vi "Read Comments.vi"(8 "error in (no error)":errorcluster, 11 "Asset External Calibration in":refnum<class "Asset External Calibration.lvclass">) -> (0 "error out":errorcluster, 2 "comments":string, 3 "Asset External Calibration out":refnum<class "Asset External Calibration.lvclass">)   [LabVIEW 2018, in "Asset External Calibration.lvclass"]
uses:
  Asset External Calibration.lvclass
  Asset External Calibration.lvclass/Asset External Calibration.ctl
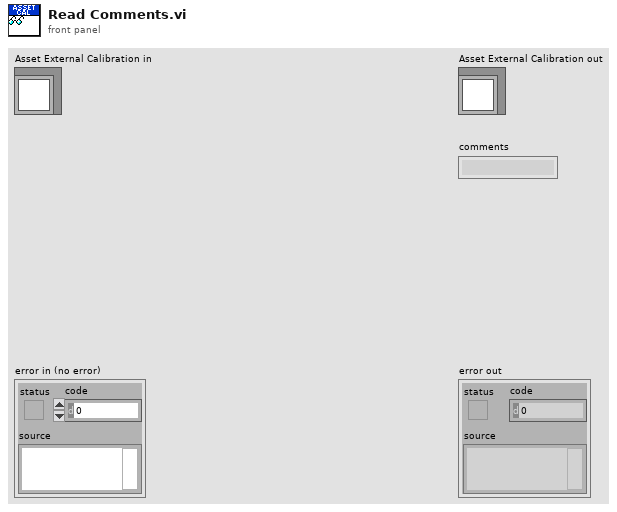
[diagram p1: front panel]
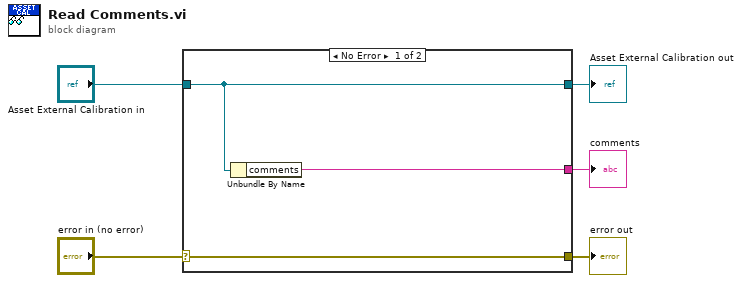
[diagram p0: block diagram]
diagram:
  n1 = case shown="No Error" "error in (no error)" {
    selector: "error in (no error)" -> [w8 w9]
    tunnel: [w8 w9] -> w4
    tunnel: [w7 w10] -> w2
    tunnel: "Asset External Calibration in" -> [w7 w10]
    tunnel: [w6 _] -> w1
    frame No Error {
      n2 = Unbundle By Name(w7) -> ("comments"=w6:string)
    }
    frame Error {
    }
  }
  "error out" <- w4
  "Asset External Calibration out" <- w2
  "comments" <- w1
